vi "Assign 3 Electronic Lock (1).vi"() -> ()   [LabVIEW 2021]
panel:
  out "Y":bool
  in  "D":bool
  in  "C":bool
  in  "B":bool
  in  "A":bool
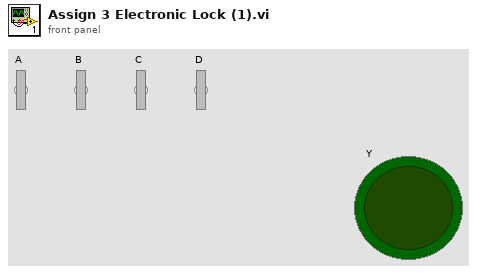
[diagram p1: front panel]
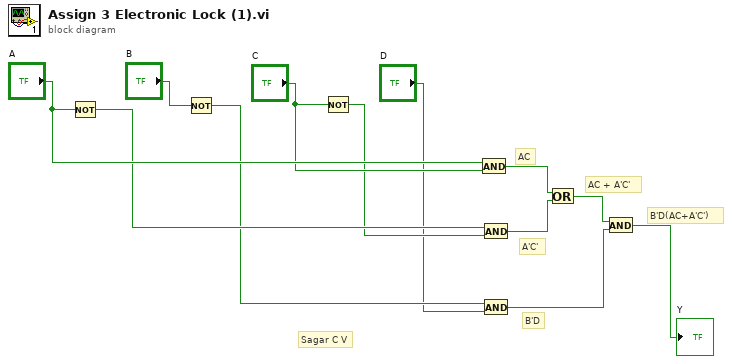
[diagram p0: block diagram]
diagram:
  # "Sagar C V"
  # "B'D(AC+A'C')"
  # "AC + A'C'"
  # "B'D"
  # "A'C'"
  # "AC"
  n1 = Not(x="A") -> (.not. x?=w4:bool)
  n2 = Not(x="B") -> (.not. x?=w2:bool)
  n3 = Not(x="C") -> (.not. x?=w3:bool)
  n4 = And(x="A", y="C") -> (x .and. y?=w7:bool)
  n5 = And(x=w4, y=w3) -> (x .and. y?=w8:bool)
  n6 = And(x=w2, y="D") -> (x .and. y?=w9:bool)
  n7 = Or(x=w7, y=w8) -> (x .or. y?=w10:bool)
  n8 = And(x=w10, y=w9) -> (x .and. y?=→"Y":bool)
